vi "Position Error.vi"(10 "Ball Data in":T1, 11 "Waypoints":i32[][](array[numeric])) -> (1 "Y Error":dbl, 2 "X Error":dbl, 3 "Next Waypoint":i32[](array[numeric]))   [LabVIEW 2012]
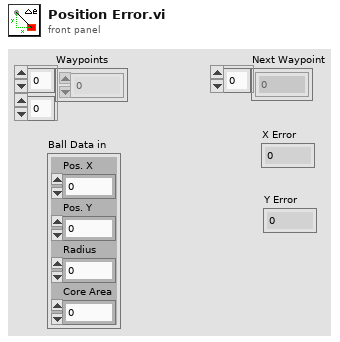
[diagram p1: front panel]
types:
  T1 = cluster{"Pos. X":i32, "Pos. Y":i32, "Radius":i32, "Core Area":i32}
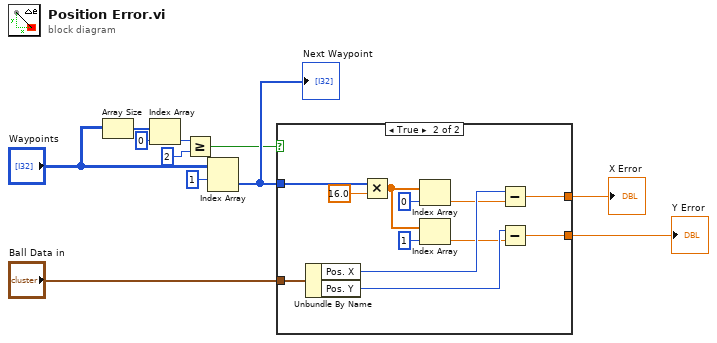
[diagram p0: block diagram]
diagram:
  n1 = Array Size(array="Waypoints") -> (size(s)=w9:i32[])
  n2 = Index Array(array=w9, index=0) -> (element=w7:i32)
  n3 = Greater Or Equal?(x=w7, y=2) -> (x >= y?=w1:bool)
  n4 = Index Array(array="Waypoints", index (row)=1) -> (element=w3:i32[])  [unwired: 1 in]
  "Next Waypoint" <- w3
  n5 = case shown="True" w1 {
    tunnel: "Ball Data in" -> [_ w23]
    tunnel: [_ w22] -> w5
    tunnel: [_ w21] -> w4
    tunnel: w3 -> [_ w17]
    frame False {
    }
    frame True {
      n6 = Unbundle By Name(w23) -> ("Pos. X"=w15:i32, "Pos. Y"=w13:i32)
      n7 = Multiply(x=w17, y=16.0) -> (x*y=w20:dbl[])
      n8 = Index Array(array=w20, index=0) -> (element=w14:dbl)
      n9 = Index Array(array=w20, index=1) -> (element=w12:dbl)
      n10 = Subtract(x=w15, y=w14) -> (x-y=w22:dbl)
      n11 = Subtract(x=w13, y=w12) -> (x-y=w21:dbl)
    }
  }
  "X Error" <- w5
  "Y Error" <- w4
